vi "ReadBoolean.vi"(8 "error in (no error)":errorcluster, 10 "Key":string, 11 "GCMConfigurationManager in":refnum<class "GCMConfigurationManager.lvclass">) -> (0 "error out":errorcluster, 2 "Value":bool, 3 "GCMConfigurationManager out":refnum<class "GCMConfigurationManager.lvclass">)   [LabVIEW 2014, in "GCMConfigurationManager.lvclass"]
uses:
  GCMConfigurationManager.lvclass
  GCMSection.vi
  <vilib>/Utility/config.llb/Read Key (Boolean).vi
  <vilib>/Utility/config.llb/NI_LVConfig.lvlib
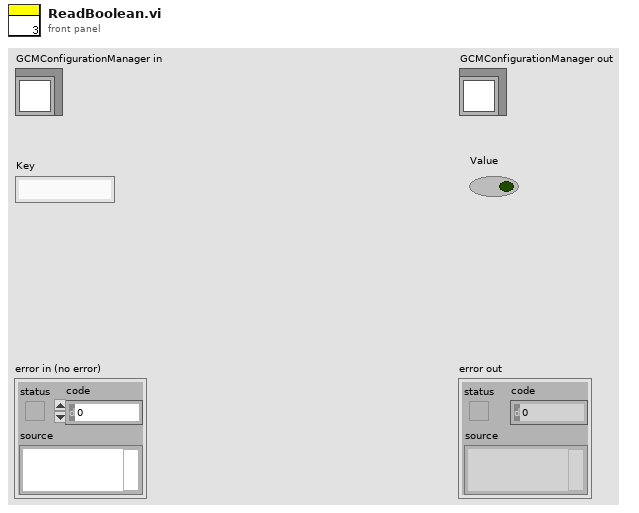
[diagram p1: front panel]
types:
  T1 = typedef "NI_LVConfig.lvlib/Config Data RefNum.ctl" = refnum<k1>
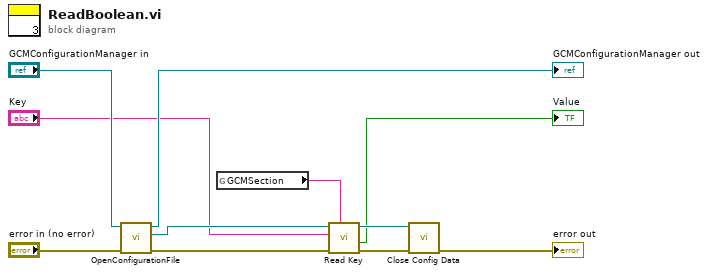
[diagram p0: block diagram]
diagram:
  n1 = call "OpenConfigurationFile.vi"("error in (no error)"="error in (no error)", "GCMConfigurationManager in"="GCMConfigurationManager in") -> ("error out"=w8:errorcluster, "FileRefnum"=w7:T1, "GCMConfigurationManager out"=→"GCMConfigurationManager out":refnum<class "GCMConfigurationManager.lvclass">)  [unwired: 7 in]
  n2 = global read "GCMSection.vi" "GCMSection"() -> (w2:string)
  n3 = call-poly <vilib>:"Read Key.vi"("section"=w2, "error in (no error)"=w8, "key"="Key", "refnum"=w7) -> ("error out"=w6:errorcluster, "value"=→"Value":bool, "refnum out"=w4:T1)  [unwired: 4 in, 1 out]
  n4 = call <vilib>:"Close Config Data.vi"("error in (no error)"=w6, "refnum"=w4) -> ("error out"=→"error out":errorcluster)  [unwired: 8 in, 1 out]
